vi "Encode Tag.vi"(1 "Wire Type":T1, 2 "ID":u64) -> (0 "Tag":u32)   [LabVIEW 2020, in "Protobuf RAW.lvlib"]
uses:
  Protobuf RAW.lvlib
  Type Serializer/Wire Type.ctl
  Wire Type Group/Wire Type Group.lvclass
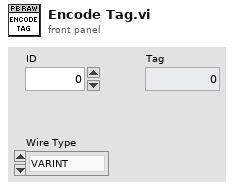
[diagram p1: front panel]
types:
  T1 = typedef "Protobuf RAW.lvlib/Wire Type Group.lvclass/Wire Type.ctl" = enum16{"VARINT", "I64", "LEN", "SGROUP", "EGROUP", "I32"}
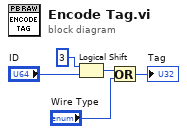
[diagram p0: block diagram]
diagram:
  n1 = Logical Shift(y=i16 3, x="ID") -> (x << y=w3:u64)
  n2 = Or(x=w3, y="Wire Type") -> (x .or. y?=→"Tag":u64)
